vi "2 DirectionChangeGoodness.vi"(1 "Test Heading":dbl) -> (0 "Goodness":dbl)   [LabVIEW 2011]
doc: "The DirectionChangeGoodness VI outputs a value between 1 and 0 that represents the goodness of the hypothetical heading from the perspective of turning as little as possible."
uses:
  2 Globals/2 Global.vi
  2 Typedefs/heading.ctl
panel:
  out "Current Heading":T1 format="%05.1f"
  # "TODO:\nThis VI could be made better to account for the wind (i.e. crossing the wind head on is less favorable)"
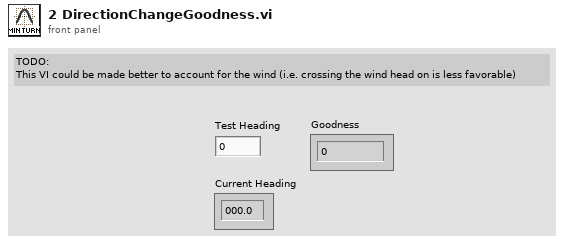
[diagram p1: front panel]
types:
  T1 = typedef "heading.ctl" = dbl
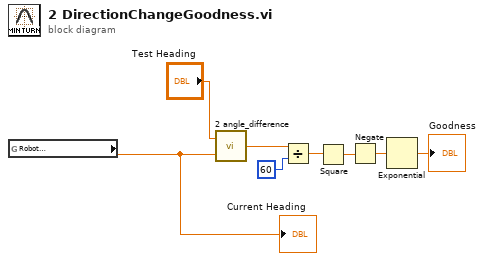
[diagram p0: block diagram]
diagram:
  n1 = global read "2 Global.vi" "Robot\nHeading"() -> (w4:T1)
  "Current Heading" <- w4
  n2 = call "2 angle_difference.vi"("Angle 2"=w4, "Angle 1"="Test Heading") -> ("Difference"=w3:dbl)
  n3 = Divide(x=w3, y=60) -> (x/y=w1:dbl)
  n4 = Square(x=w1) -> (x^2=w6:dbl)
  n5 = Negate(x=w6) -> (-x=w7:dbl)
  n6 = Exponential(1:w7) -> (0:→"Goodness":dbl)
